vi "Delete Outdated Logs.vi"(8 "error in (no error)":errorcluster, 11 "file handler in":refnum<class "File Handler.lvclass">) -> (0 "error out":errorcluster)   [LabVIEW 2024, in "Logging.lvlib" / "File Handler.lvclass"]
uses:
  File Handler.lvclass
  File Handler.lvclass/File Handler.ctl
panel:
  # "Connector Pane"
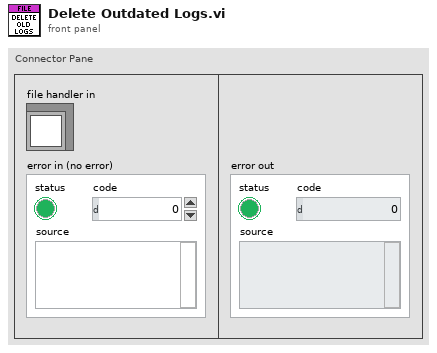
[diagram p1: front panel]
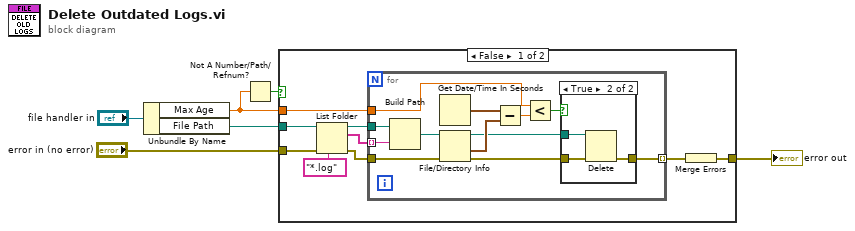
[diagram p0: block diagram]
diagram:
  n1 = Unbundle By Name("file handler in") -> ("Max Age"=w1:dbl, "File Path"=w4:path)
  n2 = Not A Number/Path/Refnum?(number/path/refnum=w1) -> (NaN/Path/Refnum?=w2:bool)
  n3 = case shown="False" w2 {
    tunnel: [w15 w32] -> w6
    tunnel: "error in (no error)" -> [w14 w32]
    tunnel: w4 -> [w11 _]
    tunnel: w1 -> [w10 _]
    frame False {
      n4 = List Folder(path=w11, pattern="*.log", error in=w14) -> (path out=w9:path, filenames=w8:string[], error out=w12:errorcluster)  [unwired: 1 in, 1 out]
      n5 = for {
        tunnel: w8 -> [w26] mode=indexing
        tunnel: w9 -> [w27]
        tunnel: w10 -> [w18]
        tunnel: w12 -> [w21]
        tunnel: [w20] -> w13 mode=indexing
        n6 = Build Path(base path=w27, name or relative path=w26) -> (appended path=w25:path)
        n7 = Get Date/Time In Seconds() -> (seconds since 1Jan1904=w19:timestamp)
        n8 = File/Directory Info(path=w25, error in=w21) -> (path out=w23:path, last mod=w24:timestamp, error out=w22:errorcluster)  [unwired: 4 out]
        n9 = Subtract(x=w19, y=w24) -> (x-y=w17:dbl)
        n10 = Less?(x=w18, y=w17) -> (x < y?=w16:bool)
        n11 = case shown="True" w16 {
          tunnel: w23 -> [_ w31]
          tunnel: w22 -> [w28 w30]
          tunnel: [w28 w29] -> w20
          frame False {
          }
          frame True {
            n12 = Delete(path (use dialog)=w31, error in=w30) -> (error out=w29:errorcluster)  [unwired: 3 in, 2 out]
          }
        }
      }
      n13 = Merge Errors(w13) -> (w15:errorcluster)
    }
    frame True {
    }
  }
  "error out" <- w6
